vi "建模板.vi"() -> ()   [LabVIEW 2016]
uses:
  <vilib>/vision/NI_Vision_Development_Module.lvlib
panel:
  in  "Exit":bool
  in  "Save":bool
  in  "Match":bool
  in  "Create Template":bool
  out "Template  Image":T1(plugin-control)
  out "Source  Image":T1(plugin-control)
  # "建立模板界面"
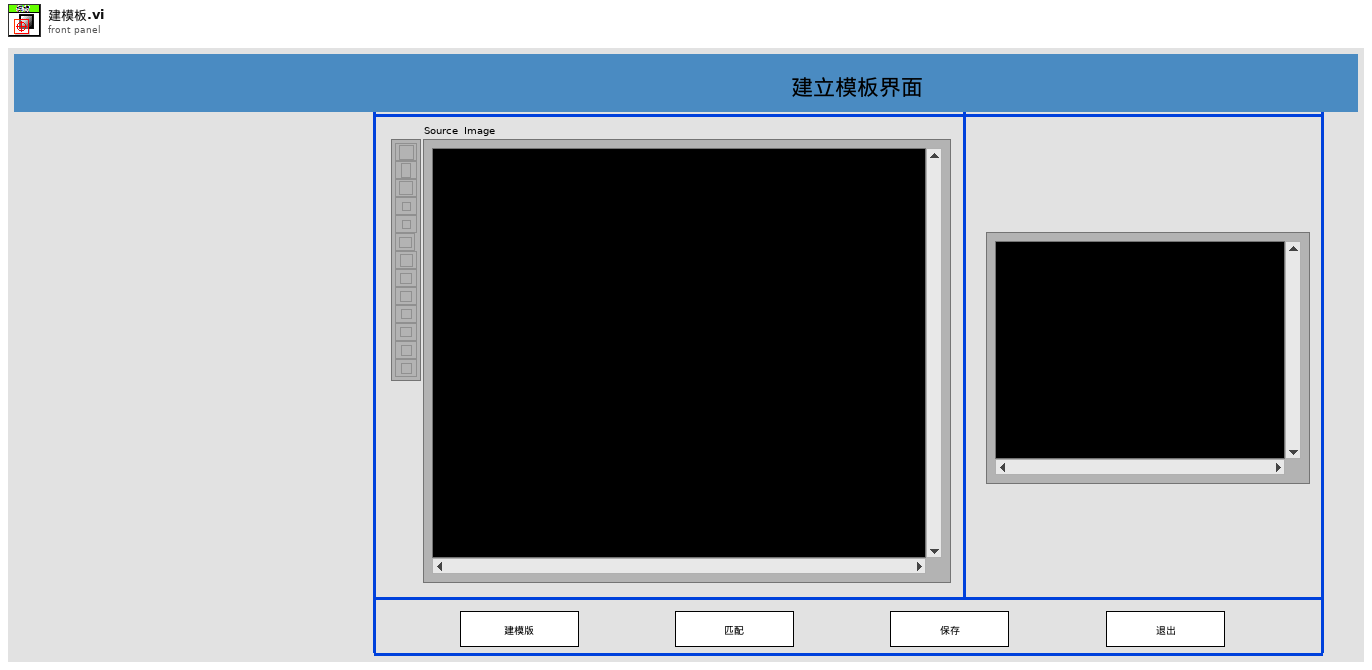
[diagram p1: front panel]
types:
  T1 = typedef "IMAQ Image.ctl" = refnum<image>
  T2 = enum8{"Enabled", "Disabled", "Disabled and Grayed Out"}
  T3 = cluster{"Algorithm":i32, "Number of Matches Requested":i32, "Minimum Match Score":sgl, "SubPixel Accuracy":bool, "Rotation Angle Ranges":cluster{"Start":sgl, "End":sgl}[], "Show Search Area":bool, "Show Result":bool}
  T4 = cluster{"Global Rectangle":i32[], "Contours":cluster{"Contour Type":u32, "ROI Type":u32, "Points":i32[]}[]}
  T5 = cluster{"Position":cluster{"x":sgl, "y":sgl}, "Angle":sgl, "Scale":sgl, "Score":sgl, "Bounding Box":cluster{"x":sgl, "y":sgl}[]}[]
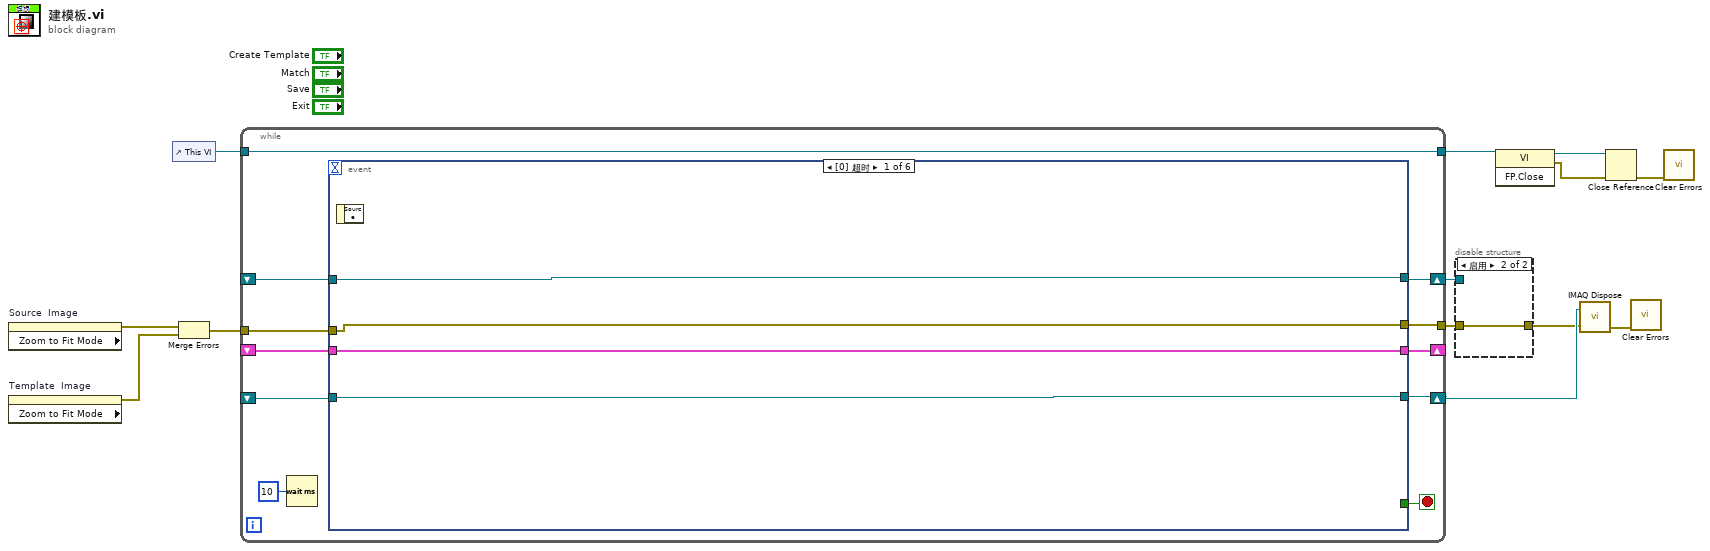
[diagram p0: block diagram]
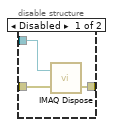
[diagram p2: hidden frame]
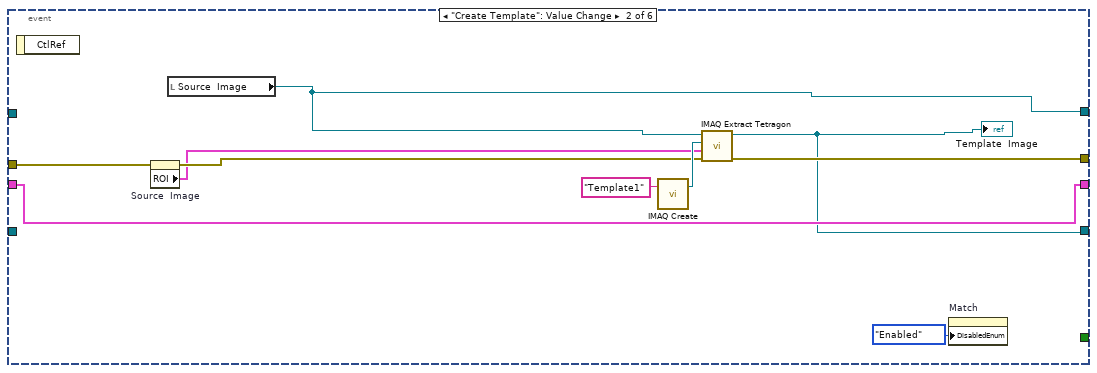
[diagram p3: hidden frame]
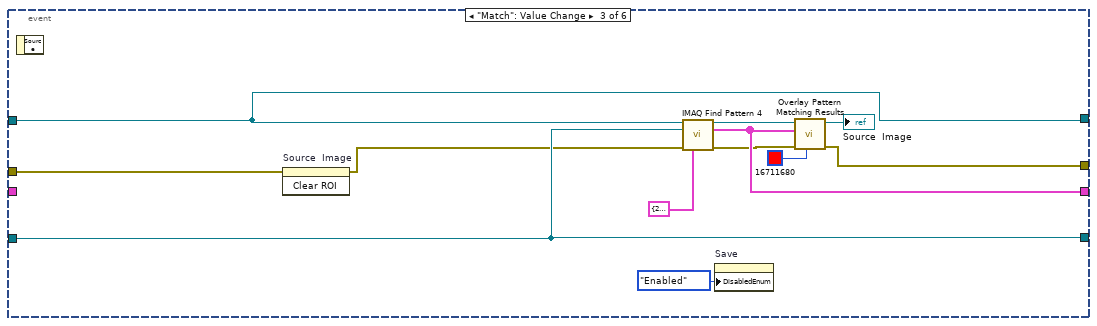
[diagram p4: hidden frame]
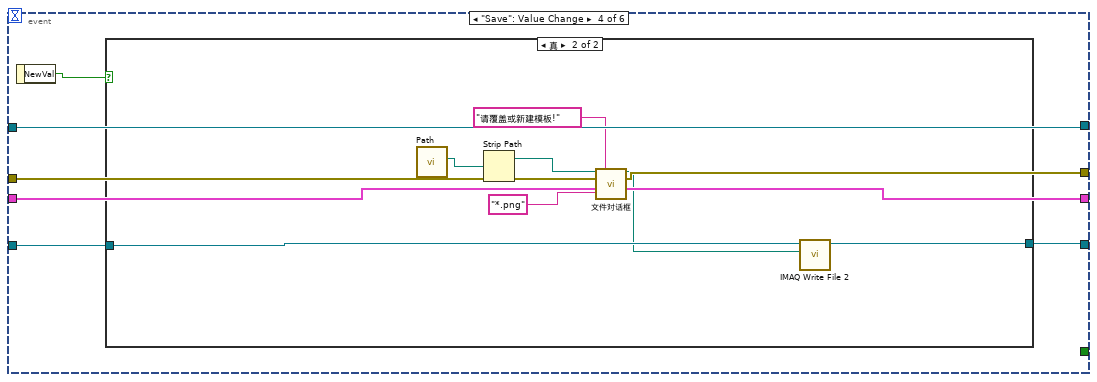
[diagram p5: hidden frame]
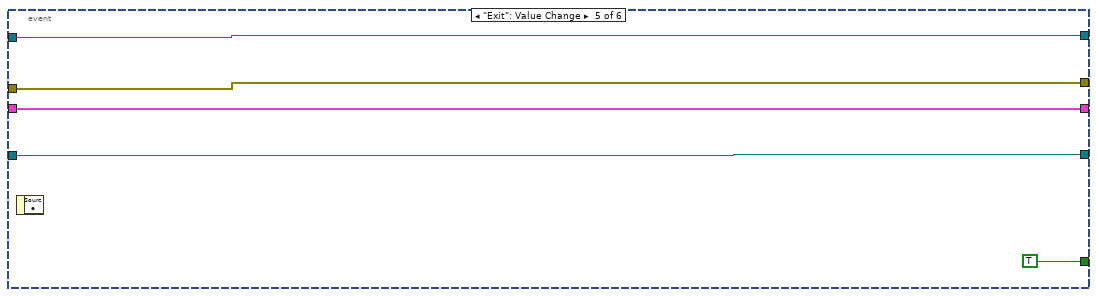
[diagram p7: hidden frame]
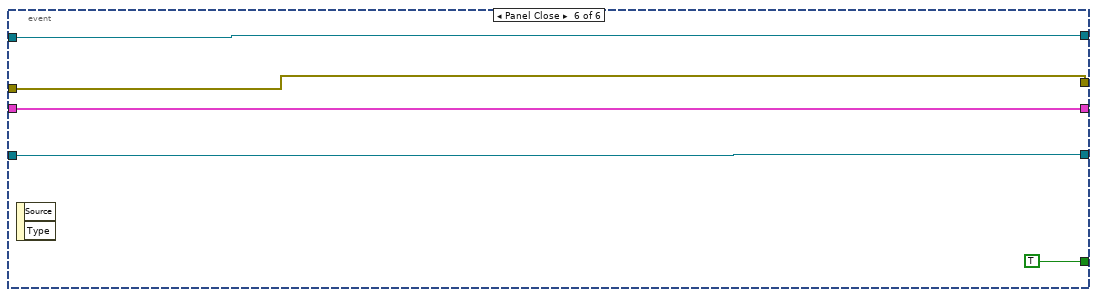
[diagram p8: hidden frame]
diagram:
  n1 = property on="Source  Image" class="ImageControl" props=["Zoom to Fit Mode"]() -> (error out=w2:errorcluster)  [unwired: 2 in, 2 out]
  n2 = property on="Template  Image" class="ImageControl" props=["Zoom to Fit Mode"]() -> (error out=w3:errorcluster)  [unwired: 2 in, 2 out]
  n3 = control-ref of="This VI"() -> (w9:refnum<vi>)
  n4 = Merge Errors(w2, w3) -> (w1:errorcluster)
  n5 = while {
    tunnel: [w22] -> w12
    shift-right: [w21] -> w13
    shift-left: _ -> [w20]
    tunnel: w9 -> [w19]
    tunnel: [w19] -> w8
    shift-right: [w18] -> w4
    shift-left: _ -> [w17]
    shift-right: [w16] -> _
    shift-left: _ -> [w15]
    tunnel: w1 -> [w14]
    stop <- w23 stop-if-true
    n6 = Wait (ms)(milliseconds to wait=u32 10) -> ()  [unwired: 1 out]
    n7 = event shown="[0] 超时" {
      selector: _ -> [_ _ _ _ _ _]
      dyn-events: _ -> [_ _ _ _ _ _]
      timeout: _ -> [_ _ _ _ _ _]
      tunnel: w17 -> [w27 _ w43 w54 w67 w72]
      tunnel: [_ _ _ _ TRUE TRUE] -> w23
      tunnel: [w26 w38 w46 w53 w66 w71] -> w22
      tunnel: [w28 w29 w42 w55 w68 w74] -> w21
      tunnel: w20 -> [w28 _ w42 w56 w68 w74]
      tunnel: w14 -> [w26 w32 w40 w53 w66 w71]
      tunnel: [w27 w33 w43 w54 w67 w72] -> w18
      tunnel: [w25 w36 w48 w52 w65 w70] -> w16
      tunnel: w15 -> [w25 w36 _ w52 w65 w70]
      event Timeout {
        n8 = event-data() -> ()  [unwired: 1 in, 1 out]
      }
      event "Create Template": Value Change {
        n9 = event-data() -> ()  [unwired: 1 in, 1 out]
        n10 = property on="Source  Image" class="ImageControl"(error in=w32) -> (error out=w31:errorcluster, "ROI"=w30:T4)  [unwired: 1 in, 1 out]
        n11 = local read "Source  Image"() -> (w33:T1)
        n12 = call "IMAQ Create"("Image Name"="Template1") -> ("New Image"=w34:T1)  [unwired: 4 in, 1 out]
        n13 = call-poly "IMAQ Extract Tetragon"("error in (no error)"=w31, "ROI Descriptor"=w30, "Image Dst"=w34, "Image Src"=w33) -> ("error out"=w38:errorcluster, "Image Dst Out"=w29:T1)  [unwired: 6 in]
        "Template  Image" <- w29
        n14 = property on="Match" class="Bool (严格)"("DisabledEnum"=T2."Enabled" ("Disabled")) -> ()  [unwired: 2 in, 2 out]
      }
      event "Match": Value Change {
        n15 = event-data() -> ()  [unwired: 1 in, 1 out]
        n16 = invoke on="Source  Image" class="ImageControl" method="Clear ROI"(error in=w40) -> (error out=w39:errorcluster)  [unwired: 2 in, 2 out]
        n17 = call "IMAQ Find Pattern 4"("Image"=w43, "Template"=w42, "error in"=w39, "Settings"=T3 {"Algorithm"=2, "Number of Matches Requested"=2, "Minimum Match Score"=600.0, "SubPixel Accuracy"=TRUE, "Rotation Angle Ranges"=[{"Start"=-20.0, "End"=20.0}], "Show Search Area"=FALSE, "Show Result"=TRUE}) -> ("Image Out"=w49:T1, "Matches (pixel)"=w48:T5, "error out"=w47:errorcluster)  [unwired: 5 in, 4 out]
        n18 = property on="Save" class="Bool (严格)"("DisabledEnum"=T2."Enabled" ("Disabled")) -> ()  [unwired: 2 in, 2 out]
        n19 = call "Overlay Pattern Matching Results.vi"("Color"=u32 16711680, "error in"=w47, "Matches"=w48, "Image"=w49) -> ("error out"=w46:errorcluster, "Image Out"=→"Source  Image":T1)  [unwired: 6 in]
      }
      event "Save": Value Change {
        n20 = event-data() -> ("NewVal"=w51:bool)  [unwired: 1 in]
        n21 = case shown="真" w51 {
          tunnel: w56 -> [w57 w64]
          tunnel: [w57 w63] -> w55
          frame False {
          }
          frame True {
            n22 = call "Path.vi"() -> ("ini"=w62:path)  [unwired: 11 in]
            n23 = Strip Path(path=w62) -> (stripped path=w61:path)  [unwired: 1 out]
            n24 = call "文件对话框"("start path"=w61, "prompt"="请覆盖或新建模板!", "pattern (all files)"="*.png") -> ("selected path"=w58:path)  [unwired: 9 in, 3 out]
            n25 = call-poly "IMAQ Write File 2"("File Path"=w58, "Image"=w64) -> ("Image Out (duplicate)"=w63:T1)  [unwired: 8 in, 1 out]
          }
        }
      }
      event "Exit": Value Change {
        n26 = event-data() -> ()  [unwired: 1 in, 1 out]
      }
      event Panel Close {
        n27 = event-data() -> ()  [unwired: 1 in, 2 out]
      }
    }
  }
  n28 = disable-structure shown="启用" {
    disable-tunnel: w12 -> [w77 w78]
    disable-tunnel: [w76 w78] -> w11
    disable-tunnel: w4 -> [w75 _]
    frame Disabled {
      n29 = call "IMAQ Dispose"("Image"=w75, "error in (no error)"=w77) -> ("error out"=w76:errorcluster)  [unwired: 4 in]
    }
    frame Enabled {
    }
  }
  n30 = invoke class="VI" method="FP.Close"(reference=w8) -> (reference out=w7:refnum<vi>, error out=w6:errorcluster)  [unwired: 2 in, 1 out]
  n31 = call "IMAQ Dispose"("Image"=w13, "error in (no error)"=w11) -> ("error out"=w10:errorcluster)  [unwired: 4 in]
  n32 = Close Reference(reference=w7, error in (no error)=w6) -> (error out=w5:errorcluster)
  n33 = call <vilib>:"Clear Errors.vi"("error in (no error)"=w10) -> ()  [unwired: 5 in, 2 out]
  n34 = call <vilib>:"Clear Errors.vi"("error in (no error)"=w5) -> ()  [unwired: 5 in, 2 out]
